vi "SmartSEM Remote API goto min or max FIB probe current.vi"(8 "error in":errorcluster, 9 "Min or Max":string(combo)="Min", 10 "FIB Probe":string(combo), 11 "ActiveX Container":refnum<k7>(container)) -> (2 "Goto probe":string, 3 "reference out":refnum<k7>)   [LabVIEW 2018]
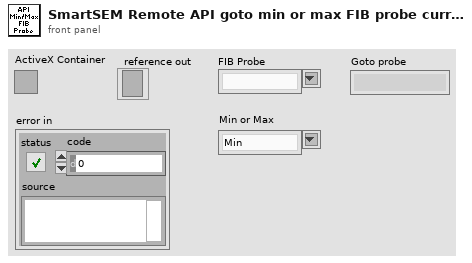
[diagram p1: front panel]
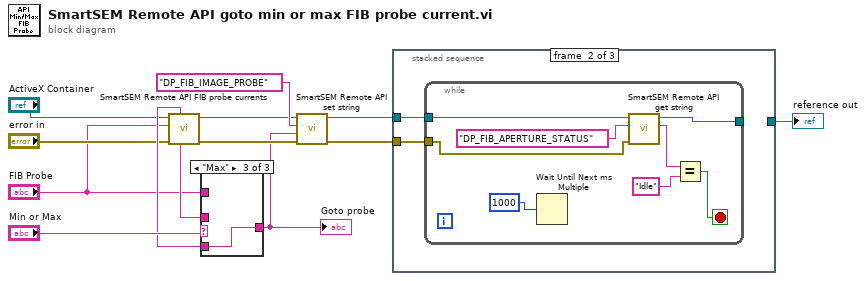
[diagram p0: block diagram]
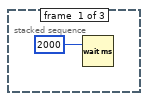
[diagram p2: hidden frame]
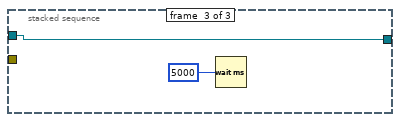
[diagram p3: hidden frame]
diagram:
  n1 = call "SmartSEM Remote API FIB probe currents.vi"("error in"="error in", "FIB Probe"="FIB Probe", "ActiveX Container"="ActiveX Container") -> ("error out"=w11:errorcluster, "reference out"=w12:refnum<k7>, "Min probe"=w9:string, "Max probe"=w8:string)  [unwired: 1 in, 4 out]
  n2 = case shown="\"Max\"" "Min or Max" {
    tunnel: w9 -> [_ w15 _]
    tunnel: w8 -> [_ _ w16]
    tunnel: [w14 w15 w16] -> w7
    tunnel: "FIB Probe" -> [w14 _ _]
    frame Default {
    }
    frame "Min" {
    }
    frame "Max" {
    }
  }
  "Goto probe" <- w7
  n3 = call "SmartSEM Remote API set string.vi"("error in"=w11, "vValue"=w7, "lpszParam"="DP_FIB_IMAGE_PROBE", "ActiveX Container"=w12) -> ("error out"=w2:errorcluster, "reference out"=w3:refnum<k7>)  [unwired: 6 in]
  n4 = stacked-sequence {
    tunnel: w3 -> [_ w19 w28]
    tunnel: [_ _ w28] -> w6
    tunnel: w2 -> [_ w18 _]
    frame #0 {
      n5 = Wait (ms)(milliseconds to wait=u32 2000) -> ()  [unwired: 1 out]
    }
    frame #1 {
      n6 = while {
        tunnel: w19 -> [w24]
        tunnel: [w23] -> _
        tunnel: w18 -> [w22]
        stop <- w25 stop-if-true
        n7 = Wait Until Next ms Multiple(millisecond multiple=u32 1000) -> ()  [unwired: 1 out]
        n8 = call "SmartSEM Remote API get string.vi"("error in"=w22, "lpszParam"="DP_FIB_APERTURE_STATUS", "ActiveX Container"=w24) -> ("data"=w21:string, "reference out"=w23:refnum<k7>)  [unwired: 6 in, 1 out]
        n9 = Equal?(x=w21, y="Idle" ("lpszParam")) -> (x = y?=w25:bool)
      }
    }
    frame #2 {
      n10 = Wait (ms)(milliseconds to wait=u32 5000) -> ()  [unwired: 1 out]
    }
  }
  "reference out" <- w6
